vi "Set Result Collector.vi"(8 "error in (no error)":errorcluster, 10 "Result Collector.lvclass":refnum<class "Result Collector.lvclass">, 11 "Report Generator in":refnum<class "Report Generator.lvclass">) -> (0 "error out":errorcluster, 3 "Report Generator out":refnum<class "Report Generator.lvclass">)   [LabVIEW 2020, in "Report Generator.lvclass"]
uses:
  Report Generator.lvclass
  Result Collector/Result Collector.lvclass
  Report Generator.lvclass/Report Generator.ctl
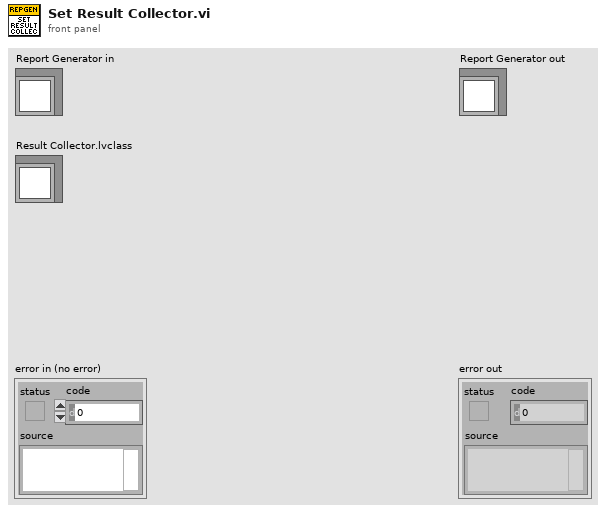
[diagram p1: front panel]
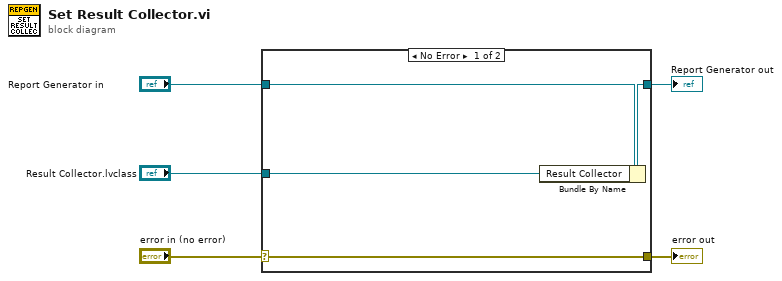
[diagram p0: block diagram]
diagram:
  n1 = case shown="No Error" "error in (no error)" {
    selector: "error in (no error)" -> [w9 w10]
    tunnel: [w9 w10] -> w4
    tunnel: [w7 w11] -> w2
    tunnel: "Report Generator in" -> [w8 w11]
    tunnel: "Result Collector.lvclass" -> [w6 _]
    frame No Error {
      n2 = Bundle By Name(cluster=w8, "Result Collector"=w6) -> (w7:refnum<class "Report Generator.lvclass">)
    }
    frame Error {
    }
  }
  "error out" <- w4
  "Report Generator out" <- w2
